vi "InitChannels.vi"(8 "error in (no error)":errorcluster, 11 "config in":T3) -> (0 "error out":errorcluster, 2 "register trends":T1[](array[typedef]), 3 "config out":T3)   [LabVIEW 2017, in "ModbusMaster.lvlib"]
uses:
  <vilib>/addons/InsightCM/Devices/Shared/Common/ModbusMaster/ModbusMaster.lvlib
  <vilib>/addons/InsightCM/Devices/Shared/Common/ModbusMaster/controls/config.ctl
  <vilib>/addons/InsightCM/Devices/Shared/Common/ModbusMaster/controls/ModbusDevice.ctl
  <vilib>/Modbus/master/Modbus Master.lvclass
  <vilib>/addons/InsightCM/Devices/Shared/Common/ModbusMaster/controls/ModbusChannel.ctl
  <vilib>/addons/InsightCM/Devices/Shared/Common/ModbusMaster/controls/RegisterType.ctl
  <vilib>/addons/InsightCM/MessageBus/Base/controls/DataSource.ctl
  <vilib>/addons/InsightCM/MessageBus/Base/controls/KeyValuePair.ctl
  <vilib>/addons/InsightCM/Devices/Shared/Common/ModbusMaster/controls/DataSourceChannel.ctl
  <vilib>/addons/InsightCM/Devices/Shared/Common/DataEventCreator/controls/RegisterTrendPoints.ctl
  <vilib>/addons/InsightCM/Devices/Shared/Common/DataEventCreator/controls/Registry_Trend.ctl
  <vilib>/addons/PointValueMap/subVIs/Point_Create_double.vi
  <vilib>/addons/InsightCM/Devices/Shared/Common/DataEventCreator/DataEventCreator.lvlib
  <vilib>/addons/InsightCM/Utilities/GlobalConfiguration/GlobalConfiguration.lvlib
  <vilib>/addons/PointValueMap/PointValueMap.lvlib
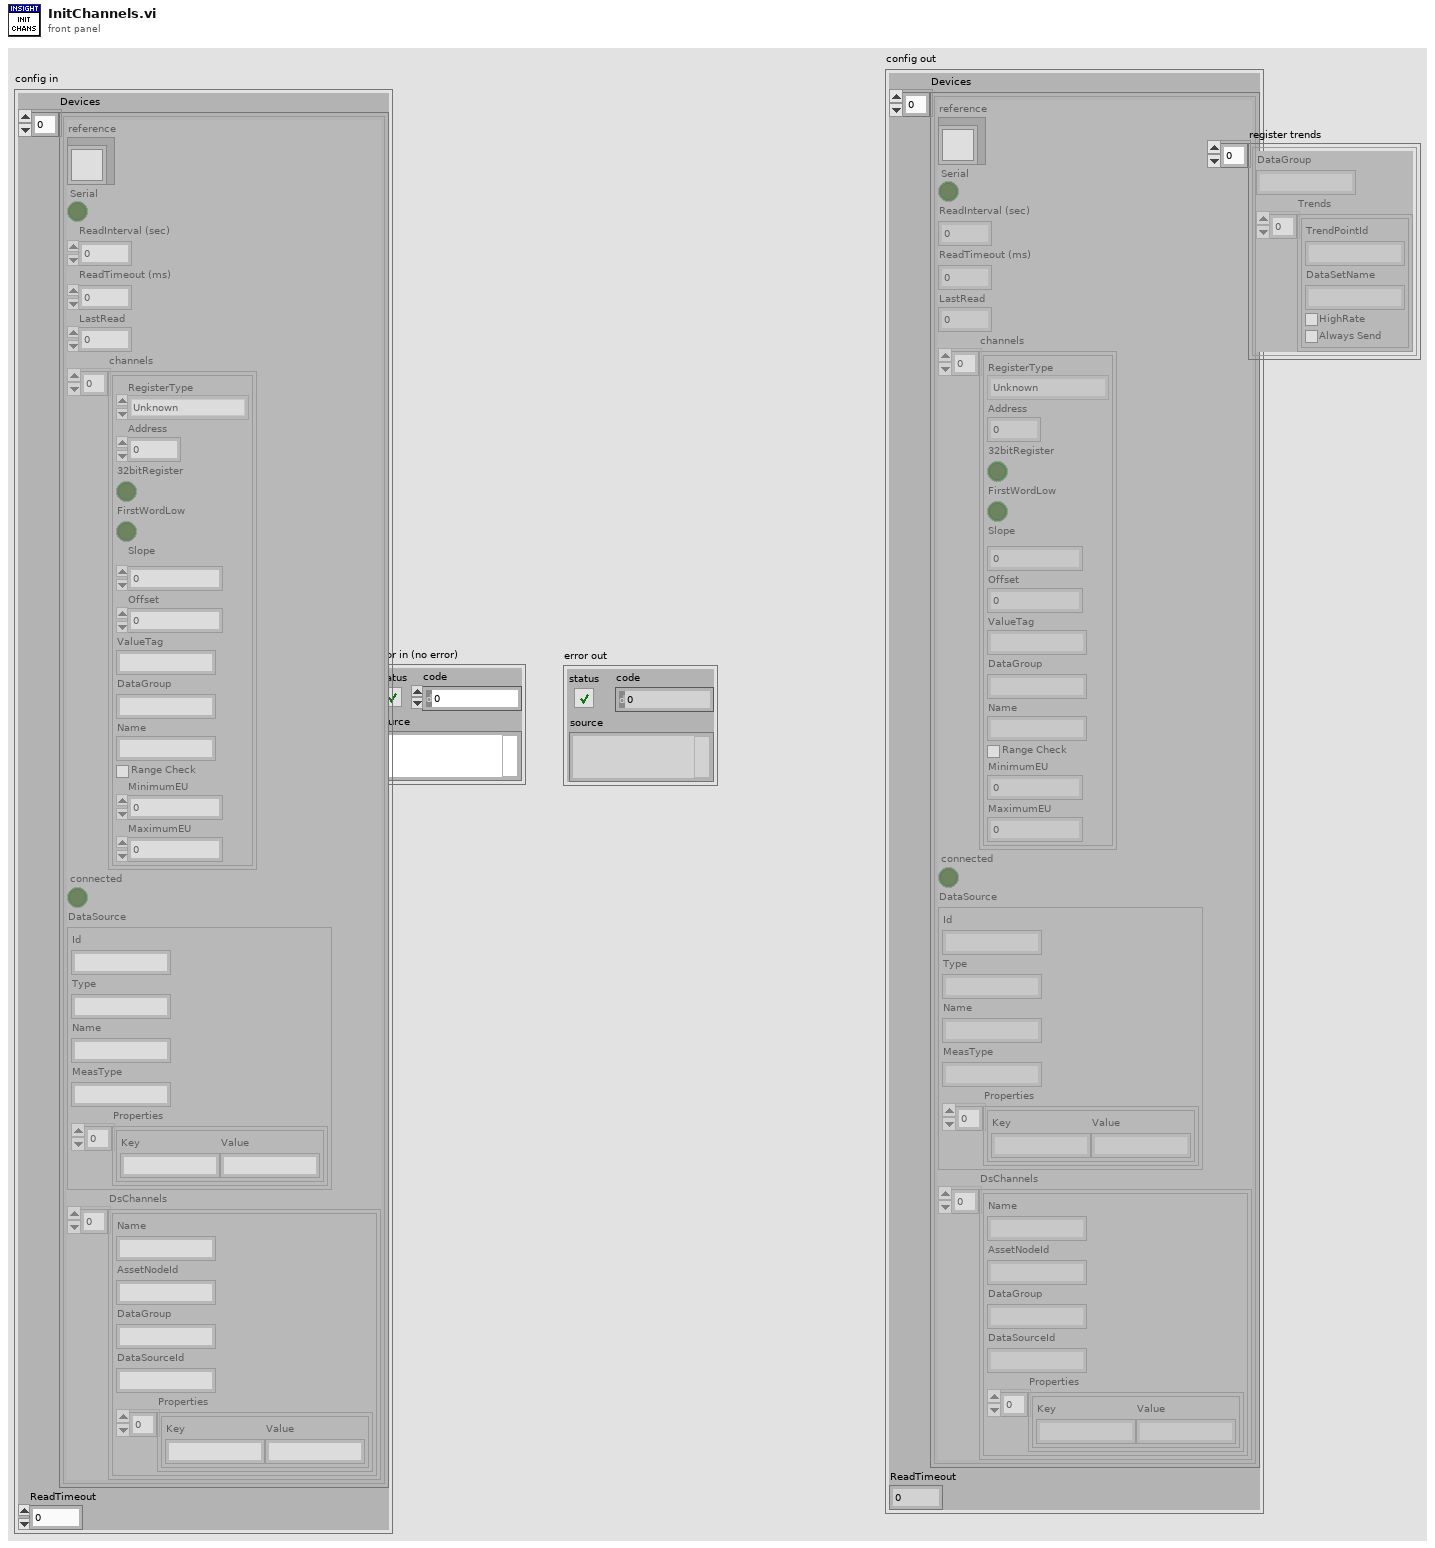
[diagram p1: front panel]
types:
  T1 = typedef "DataEventCreator.lvlib/RegisterTrendPoints.ctl" = cluster{"DataGroup":string, "Trends":T2[]}
  T2 = typedef "DataEventCreator.lvlib/Registry_Trend.ctl" = cluster{"TrendPointId":string, "DataSetName":string, "HighRate":bool, "Always Send":bool}
  T3 = typedef "ModbusMaster.lvlib/config.ctl" = cluster{"Devices":T4[], "ReadTimeout":i32}
  T4 = typedef "ModbusMaster.lvlib/ModbusDevice.ctl" = cluster{"reference":refnum<class "Modbus Master.lvclass">, "Serial":bool, "ReadInterval (sec)":dbl, "ReadTimeout (ms)":i32, "LastRead":dbl, "channels":T5[], "connected":bool, "DataSource":T7, "DsChannels":T9[]}
  T5 = typedef "ModbusMaster.lvlib/ModbusChannel.ctl" = cluster{"RegisterType":T6, "Address":i32, "32bitRegister":bool, "FirstWordLow":bool, "Slope":dbl, "Offset":dbl, "ValueTag":string, "DataGroup":string, "Name":string, "Range Check":bool, "MinimumEU":dbl, "MaximumEU":dbl}
  T6 = typedef "ModbusMaster.lvlib/RegisterType.ctl" = enum16{"Unknown", "Coil", "Discrete Input", "Holding Register", "Input Register"}
  T7 = typedef "DataSource.ctl" = cluster{"Id":string, "Type":string, "Name":string, "MeasType":string, "Properties":T8[]}
  T8 = typedef "KeyValuePair.ctl" = cluster{"Key":string, "Value":string}
  T9 = typedef "ModbusMaster.lvlib/DataSourceChannel.ctl" = cluster{"Name":string, "AssetNodeId":string, "DataGroup":string, "DataSourceId":string, "Properties":T8[]}
  T10 = typedef "PointValueMap.lvlib/PointMap.ctl" = refnum<data-value>
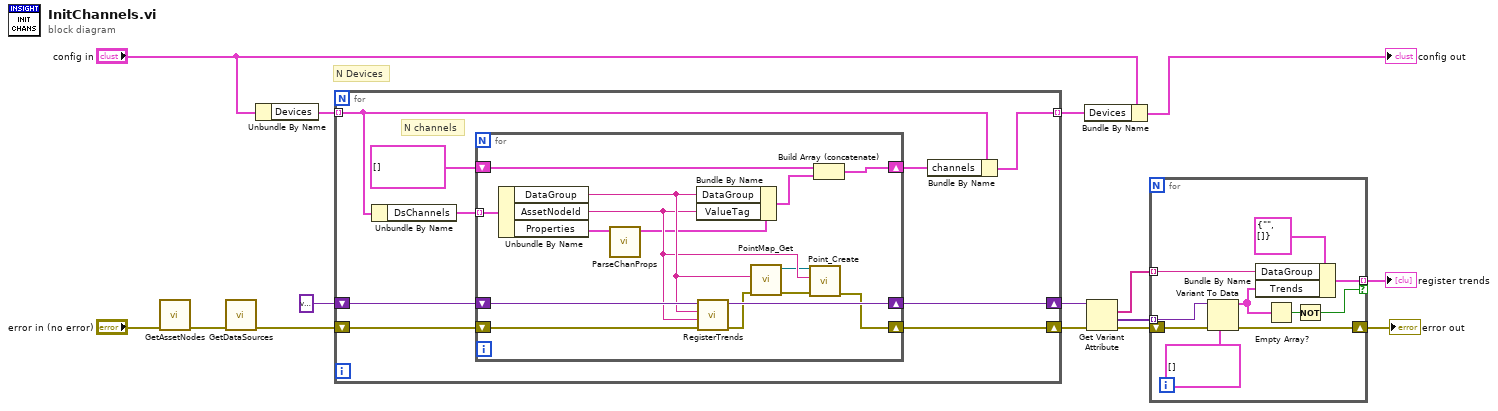
[diagram p0: block diagram]
diagram:
  # "N Devices"
  n1 = call <vilib>:"GetAssetNodes.vi"("error in (no error)"="error in (no error)") -> ("error out"=w7:errorcluster)  [unwired: 8 in, 2 out]
  n2 = call <vilib>:"GetDataSources.vi"("error in (no error)"=w7) -> ("error out"=w4:errorcluster)  [unwired: 8 in, 2 out]
  n3 = Unbundle By Name("config in") -> ("Devices"=w13:T4[])
  n4 = for {
    tunnel: w13 -> [w23] mode=indexing
    tunnel: [w20] -> w10 mode=indexing
    shift-right: [w18] -> w9
    shift-left: variant -> [w19]
    shift-right: [w17] -> w5
    shift-left: w4 -> [w16]
    # "N channels"
    n5 = Unbundle By Name(w23) -> ("DsChannels"=w24:T9[])
    n6 = for {
      tunnel: w24 -> [w39] mode=indexing
      shift-right: [w38] -> w22
      shift-left: T5[] [] -> [w37]
      shift-right: [w35] -> w18
      shift-left: w19 -> [w36]
      shift-right: [w33] -> w17
      shift-left: w16 -> [w32]
      n7 = Unbundle By Name(w39) -> ("DataGroup"=w34:string, "AssetNodeId"=w31:string, "Properties"=w25:T8[])
      n8 = call <vilib>:"ParseChanProps.vi"("properties"=w25) -> ("channel"=w30:T5)  [unwired: 9 in, 1 out]
      n9 = Bundle By Name(cluster=w30, "DataGroup"=w34, "ValueTag"=w31) -> (w29:T5)
      n10 = call <vilib>:"RegisterTrends.vi"("error in (no error)"=w32, "asset node id"=w31, "data group"=w34, "data group map"=w36) -> ("error out"=w28:errorcluster, "data group map"=w35:variant)  [unwired: 6 in]
      n11 = call <vilib>:"PointMap_Get.vi"("error in (no error)"=w28, "Name"=w34) -> ("error out"=w27:errorcluster, "Map Out"=w26:T10)  [unwired: 7 in, 1 out]
      n12 = call-poly <vilib>:"Point_Create.vi"("Error In"=w27, "Tag"=w31, "Map"=w26) -> ("Error Out"=w33:errorcluster)  [unwired: 7 in, 1 out]
      n13 = Build Array (concatenate)(w37, w29) -> (w38:T5[])
    }
    n14 = Bundle By Name(cluster=w23, "channels"=w22) -> (w20:T4)
  }
  n15 = Bundle By Name(cluster="config in", "Devices"=w10) -> (→"config out":T3)
  n16 = Get Variant Attribute(Variant=w9, error in=w5) -> (names=w2:string[], values=w8:variant[], error out=w3:errorcluster)  [unwired: 2 in, 1 out]
  n17 = for {
    tunnel: w8 -> [w44] mode=indexing
    tunnel: [w47] -> w12 mode=indexing if=w46
    tunnel: w2 -> [w42] mode=indexing
    shift-right: [w40] -> w1
    shift-left: w3 -> [w41]
    n18 = Variant To Data(error in=w41, type=T2[] [], Variant=w44) -> (data=w43:T2[], error out=w40:errorcluster)
    n19 = Bundle By Name(cluster=T1 {"DataGroup"="", "Trends"=[]} ("register trend"), "DataGroup"=w42, "Trends"=w43) -> (w47:T1)
    n20 = Empty Array?(array=w43) -> (empty?=w48:bool)
    n21 = Not(x=w48) -> (.not. x?=w46:bool)
  }
  "error out" <- w1
  "register trends" <- w12
